vi "FarFromTrajectory.vi"(9 "Project":T1, 10 "Path":dbl[][](array[numeric]), 11 "Position":dbl[](array[numeric])) -> (2 "Far from trajectory?":bool)   [LabVIEW 2023]
uses:
  Parameters_class/Project.ctl
  <vilib>/Analysis/_algsub.llb/Real Vector Norm.vi
  <vilib>/Analysis/NI_AALPro.lvlib
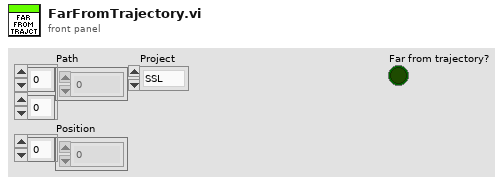
[diagram p1: front panel]
types:
  T1 = typedef "Project.ctl" = enum16{"SSL", "VSS"}
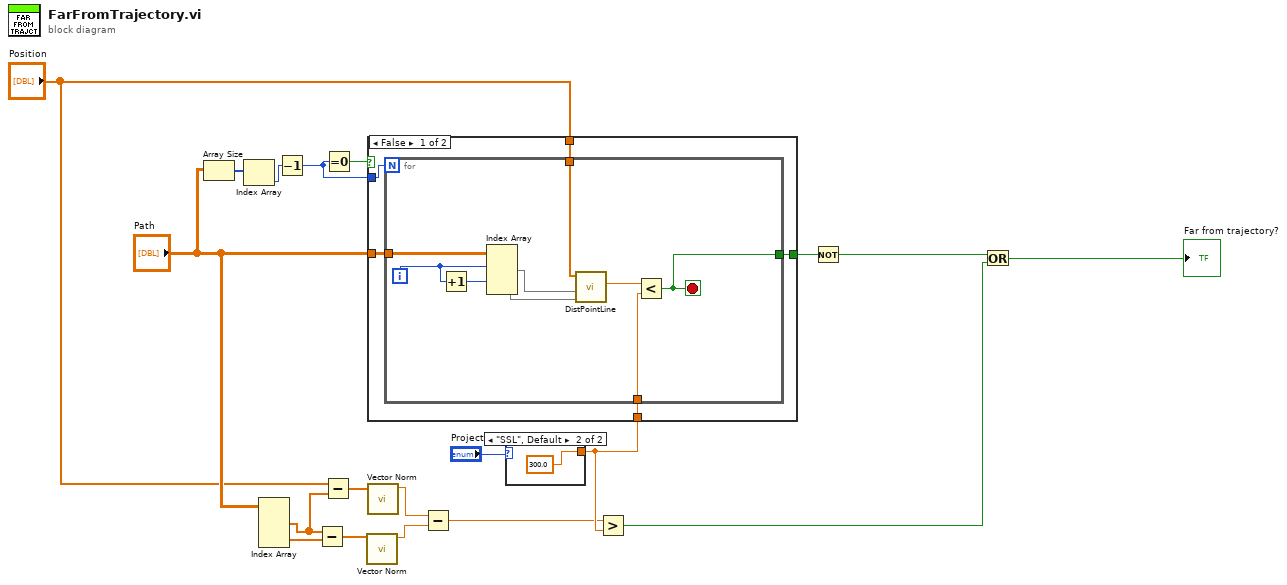
[diagram p0: block diagram]
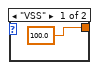
[diagram p2: hidden frame]
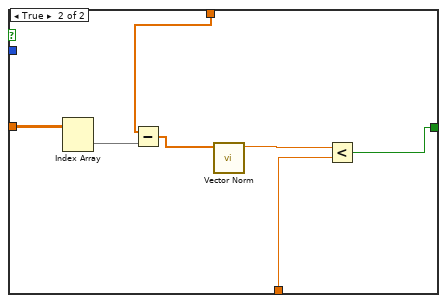
[diagram p3: hidden frame]
diagram:
  n1 = Array Size(array="Path") -> (size(s)=w19:i32[])
  n2 = Index Array(array=w19) -> (element=w18:i32)  [unwired: 1 in]
  n3 = Index Array(array="Path") -> (element #1=w11:dbl[], element #2=w13:dbl[])  [unwired: 4 in]
  n4 = Decrement(x=w18) -> (x-1=w15:i32)
  n5 = Subtract(x=w11, y=w13) -> (x-y=w12:dbl[])
  n6 = Subtract(x="Position", y=w11) -> (x-y=w9:dbl[])
  n7 = Equal To 0?(x=w15) -> (x = 0?=w16:bool)
  n8 = call-poly <vilib>:"Vector Norm.vi"("Input Vector"=w12) -> ("norm"=w6:dbl)  [unwired: 9 in, 1 out]
  n9 = call-poly <vilib>:"Vector Norm.vi"("Input Vector"=w9) -> ("norm"=w7:dbl)  [unwired: 9 in, 1 out]
  n10 = Subtract(x=w7, y=w6) -> (x-y=w5:dbl)
  n11 = case shown="\"SSL\", Default" "Project" {
    tunnel: [100.0 ("y") 300.0 ("y")] -> w8
    frame "VSS" {
    }
    frame "SSL", Default {
    }
  }
  n12 = case shown="False" w16 {
    tunnel: "Path" -> [w26 w42]
    tunnel: "Position" -> [w25 w40]
    tunnel: [w24 w37] -> w17
    tunnel: w8 -> [w23 w36]
    tunnel: w15 -> [w22 _]
    frame False {
      n13 = for {
        N: w22 -> [_]
        tunnel: w26 -> [w35]
        tunnel: w25 -> [w30]
        tunnel: [w28] -> w24
        tunnel: w23 -> [w27]
        i -> [w33]
        stop <- w28 stop-if-true
        n14 = Increment(x=w33) -> (x+1=w34:i32)
        n15 = Index Array(array=w35, index (row) #1=w33, index (row) #2=w34) -> (element #1=w32:dbl[], element #2=w31:dbl[])  [unwired: 2 in]
        n16 = call "DistPointLine.vi"("P2"=w31, "P1"=w32, "Q"=w30) -> ("distance"=w29:dbl)  [unwired: 8 in]
        n17 = Less?(x=w29, y=w27) -> (x < y?=w28:bool)
      }
    }
    frame True {
      n18 = Index Array(array=w42) -> (element=w41:dbl[])  [unwired: 2 in]
      n19 = Subtract(x=w40, y=w41) -> (x-y=w39:dbl[])
      n20 = call-poly <vilib>:"Vector Norm.vi"("Input Vector"=w39) -> ("norm"=w38:dbl)  [unwired: 9 in, 1 out]
      n21 = Less?(x=w38, y=w36) -> (x < y?=w37:bool)
    }
  }
  n22 = Greater?(x=w5, y=w8) -> (0:w2:bool)
  n23 = Not(x=w17) -> (.not. x?=w4:bool)
  n24 = Or(x=w4, y=w2) -> (x .or. y?=→"Far from trajectory?":bool)
